vi "Periodic Tasks.vi"(8 "error in":errorcluster) -> ()   [LabVIEW 2023]
doc: "This VI runs in parallel to other tasks. It can contain as many user-defined periodic loops as you need. These can carry out PID or other sorts of timed response."
uses:
  <vilib>/Rock Robotics/WPI/ThirdParty/Phoenix6/getters/GetCANcoder_AbsPosition.vi
  <vilib>/Rock Robotics/Network Tables/NT Write Number.vi
  <vilib>/Rock Robotics/Network Tables/NT Write Boolean.vi
  <vilib>/Rock Robotics/Network Tables/NT Write String.vi
  <vilib>/Rock Robotics/WPI/ThirdParty/JAS_Junk/TrajLib/Trajectory_Library.lvlib
  <vilib>/Rock Robotics/WPI/ThirdParty/PhotonVisionLib/PhotonVisionLib.lvlib
  <vilib>/Rock Robotics/Network Tables/NT Write Integer.vi
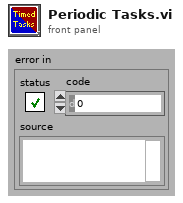
[diagram p1: front panel]
types:
  T1 = typedef "DeviceReference.ctl" = cluster{"CANbus Name":string, "Device Encoding":u32, "Device Name":string}
  T2 = cluster{"Value":dbl, "System Timestamp":dbl, "CANivore Timestamp":dbl, "ECU Timestamp":dbl}
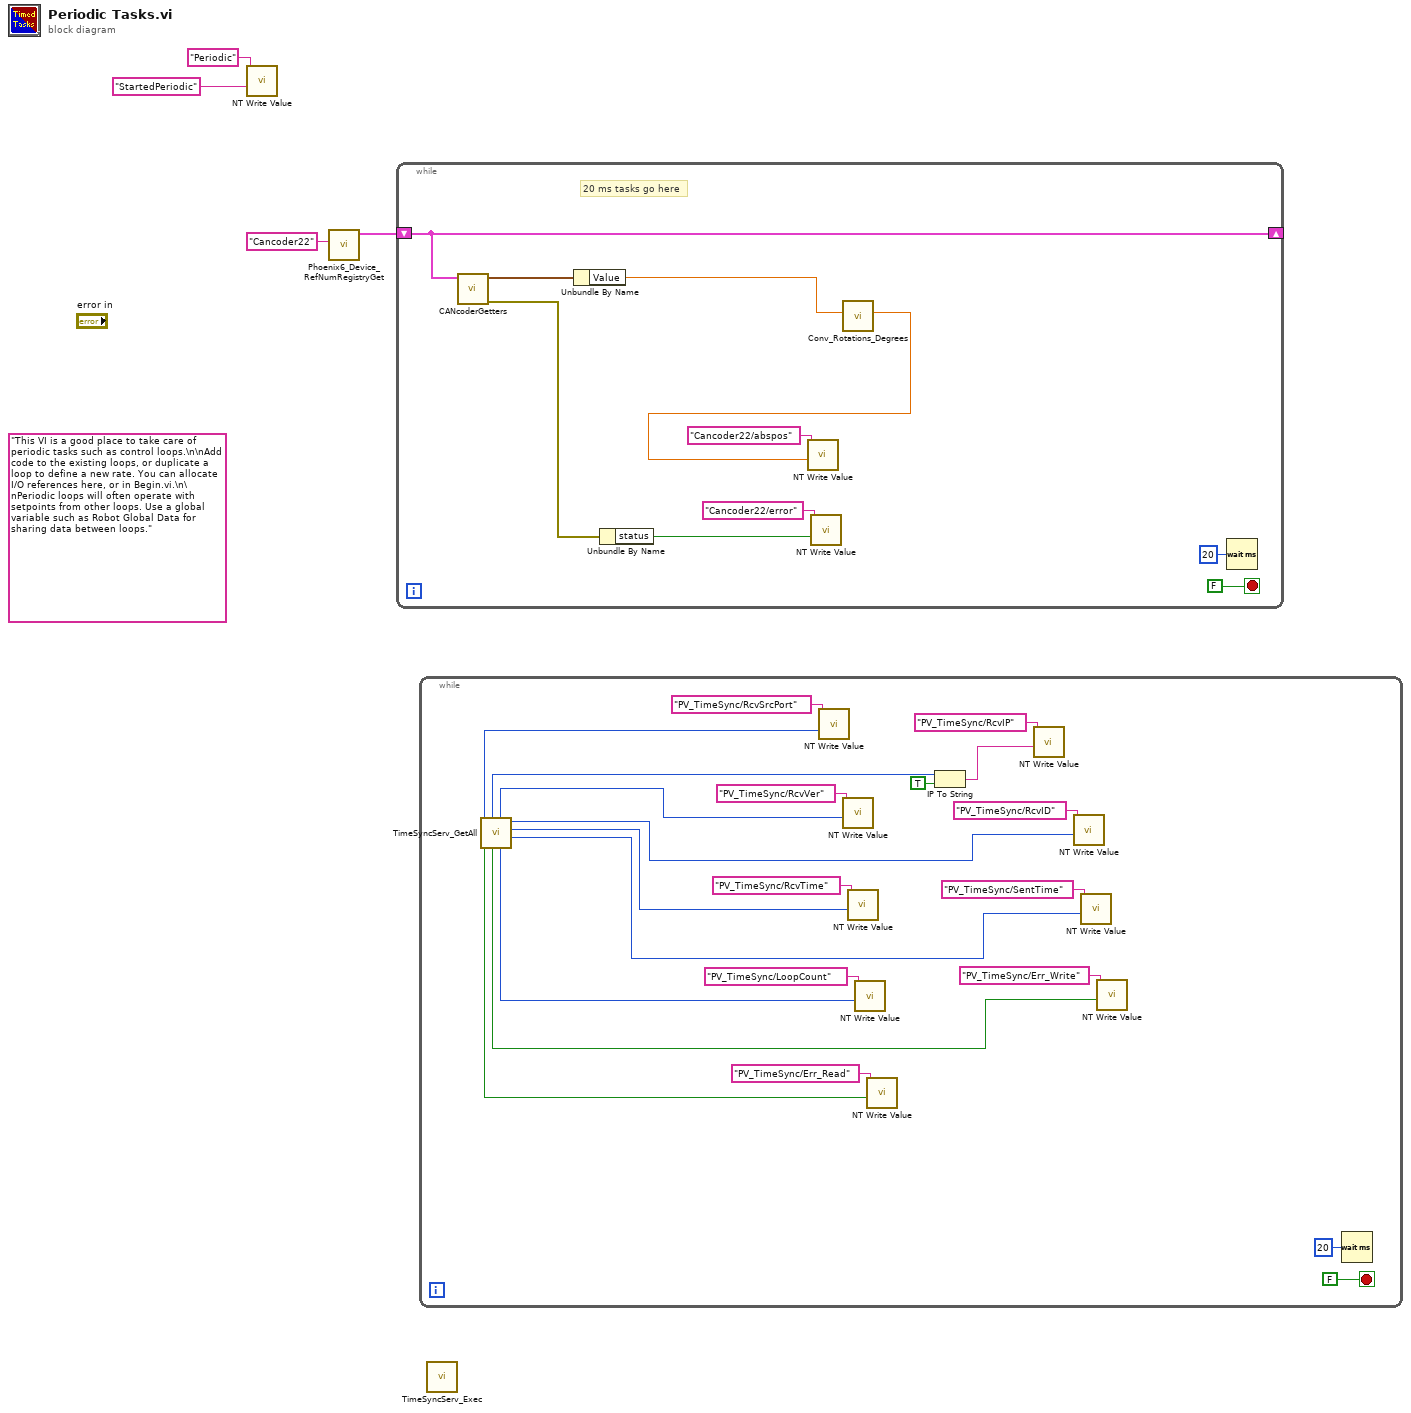
[diagram p0: block diagram]
diagram:
  (unwired) "This VI is a good place to take care of periodic tasks such as control loops.\n\nAdd code to the existing loops, or duplicate a loop to define a new rate. You can allocate I/O references here, or in Begin.vi.\n\nPeriodic loops will often operate with setpoints from other loops. Use a global variable such as Robot Global Data for sharing data between loops."
  n1 = call-poly <vilib>:"NT Write Value.vi"("value"="StartedPeriodic", "name"="Periodic") -> ()  [unwired: 9 in, 1 out]
  n2 = call <vilib>:"Phoenix6_Device_RefNumRegistryGet.vi"("refnum name"="Cancoder22") -> ("data"=w3:T1)  [unwired: 9 in, 1 out]
  n3 = while {
    shift-right: [w12] -> _
    shift-left: w3 -> [w12]
    stop <- FALSE stop-if-true
    # "20 ms tasks go here"
    n4 = call-poly <vilib>:"CANcoderGetters.vi"("DeviceReference"=w12) -> ("error out"=w8:errorcluster, "Output"=w5:T2)  [unwired: 9 in]
    n5 = Unbundle By Name(w5) -> ("Value"=w7:dbl)
    n6 = Unbundle By Name(w8) -> ("status"=w9:bool)
    n7 = call-poly <vilib>:"NT Write Value.vi"("value"=w9, "name"="Cancoder22/error") -> ()  [unwired: 9 in, 1 out]
    n8 = call <vilib>:"Conv_Rotations_Degrees.vi"("Rotations"=w7) -> ("Degrees"=w6:dbl)  [unwired: 10 in]
    n9 = call-poly <vilib>:"NT Write Value.vi"("value"=w6, "name"="Cancoder22/abspos") -> ()  [unwired: 9 in, 1 out]
    n10 = Wait (ms)(milliseconds to wait=u32 20) -> ()  [unwired: 1 out]
  }
  n11 = while {
    stop <- FALSE stop-if-true
    n12 = call <vilib>:"TimeSyncServ_GetAll.vi"() -> ("PV_TimeSyncLastSentTime"=w21:i64, "PV_TimeSyncLastRcvTim"=w23:i64, "PV_TimeSyncLastRcvId"=w25:i8, "PV_TimeSyncLoopCount"=w19:i32, "PV_TimeSyncLastRcvVer"=w27:i8, "PV_TimeSyncServWriteErr"=w17:bool, "PV_TimeSyncServRcvIP"=w31:u32, "PV_TimeSyncServReadErr"=w15:bool, "PV_TimeSyncServLastSrcPort"=w33:u32)  [unwired: 2 in, 1 out]
    n13 = call-poly <vilib>:"NT Write Value.vi"("value"=w33, "name"="PV_TimeSync/RcvSrcPort") -> ()  [unwired: 9 in, 1 out]
    n14 = call-poly <vilib>:"NT Write Value.vi"("value"=w27, "name"="PV_TimeSync/RcvVer") -> ()  [unwired: 9 in, 1 out]
    n15 = call-poly <vilib>:"NT Write Value.vi"("value"=w23, "name"="PV_TimeSync/RcvTime") -> ()  [unwired: 9 in, 1 out]
    n16 = call-poly <vilib>:"NT Write Value.vi"("value"=w19, "name"="PV_TimeSync/LoopCount") -> ()  [unwired: 9 in, 1 out]
    n17 = call-poly <vilib>:"NT Write Value.vi"("value"=w15, "name"="PV_TimeSync/Err_Read") -> ()  [unwired: 9 in, 1 out]
    n18 = IP To String(1:TRUE ("dot notation? (F)"), 2:w31) -> (0:w29:string)
    n19 = call-poly <vilib>:"NT Write Value.vi"("value"=w29, "name"="PV_TimeSync/RcvIP") -> ()  [unwired: 9 in, 1 out]
    n20 = call-poly <vilib>:"NT Write Value.vi"("value"=w25, "name"="PV_TimeSync/RcvID") -> ()  [unwired: 9 in, 1 out]
    n21 = call-poly <vilib>:"NT Write Value.vi"("value"=w21, "name"="PV_TimeSync/SentTime") -> ()  [unwired: 9 in, 1 out]
    n22 = call-poly <vilib>:"NT Write Value.vi"("value"=w17, "name"="PV_TimeSync/Err_Write") -> ()  [unwired: 9 in, 1 out]
    n23 = Wait (ms)(milliseconds to wait=u32 20) -> ()  [unwired: 1 out]
  }
  n24 = call <vilib>:"TimeSyncServ_Exec.vi"() -> ()  [unwired: 12 in]
